vi "20110512 Plotter.vi"() -> ()   [LabVIEW 2009]
uses:
  <vilib>/Utility/miscctls.llb/LVPositionTypeDef.ctl
  <vilib>/Utility/tcp.llb/UDP Multicast Read-Only Open.vi
  shared programs/MySQL/Preset Query Enum.ctl
  <userlib>/_OpenG.lib/array/array.llb/Search 1D Array (String)__ogtk.vi
  <vilib>/Utility/miscctls.llb/LVRectTypeDef.ctl
panel:
  out "Mcast Data":string
  out "ScanStart ExptName":string
  out "TDMS file path":path
  out "Y Axis Default name":string
  in  "Tab Control 2":T1(tab)
  out "parameters to get":string[][](array[string])
  out "devices to get data from":string[](array[string])
  out "Axis Name List":string[](array[string])
  out "All Devices Core Info":string[][](array[string])
  out "Position 2":T2
  out "Position":T2
  out "UDP Mcast Error":errorcluster
  out "MY IP":string
  in  "Tab Control":enum32{"Main", "ShotData", "setup"}(tab)
  in  "Y Axis 2":u16(ring) items=["FakeCam1 shot #", "FakeCam1 exposure", "FakeCam1 gain", "Shot #"]
  in  "FilePath":bool
  out "xy graph":cluster{dbl[], dbl[]}[](graph)=[{[1.0, 2.0, 3.0, 4.0, 5.0, 6.0, 7.0, 8.0, 9.0, 10.0, 11.0, 12.0, 13.0, 14.0, 15.0, 16.0, 17.0, 18.0, 19.0, 20.0, 21.0, 22.0, 23.0, 24.0, 25.0, 26.0, 27.0, 28.0, 29.0, 30.0, 31.0, 32.0, 33.0, 34.0, 35.0, 36.0, 37.0, 38.0, 39.0, 40.0, 41.0, 42.0, 43.0, 44.0, 45.0, 46.0, 47.0, 48.0, 49.0, 50.0, 51.0, 52.0, 53.0, 54.0, 55.0, 56.0, 57.0, 58.0, 59.0, 60.0, 0.0, 0.0, 0.0], [0.1, 0.1, 0.1, 0.1, 0.1, 0.1, 0.1, 0.1, 0.1, 0.1, 0.1, 0.1, 0.1, 0.1, 0.1, 0.1, 0.1, 0.1, 0.1, 0.1, 0.15, 0.15, 0.15, 0.15, 0.15, 0.15, 0.15, 0.15, 0.15, 0.15, 0.15, 0.15, 0.15, 0.15, 0.15, 0.15, 0.15, 0.15, 0.15, 0.15, 0.2, 0.2, 0.2, 0.2, 0.2, 0.2, 0.2, 0.2, 0.2, 0.2, 0.2, 0.2, 0.2, 0.2, 0.2, 0.2, 0.2, 0.2, 0.2, 0.2, 0.0, 0.0, 0.0]}, {[1.0, 2.0, 3.0, 4.0, 5.0, 6.0, 7.0, 8.0, 9.0, 10.0, 11.0, 12.0, 13.0, 14.0, 15.0, 16.0, 17.0, 18.0, 19.0, 20.0, 21.0, 22.0, 23.0, 24.0, 25.0, 26.0, 27.0, 28.0, 29.0, 30.0, 31.0, 32.0, 33.0, 34.0, 35.0, 36.0, 37.0, 38.0, 39.0, 40.0, 41.0, 42.0, 43.0, 44.0, 45.0, 46.0, 47.0, 48.0, 49.0, 50.0, 51.0, 52.0, 53.0, 54.0, 55.0, 56.0, 57.0, 58.0, 59.0, 60.0, 0.0, 0.0, 0.0], [1.0, 2.0, 3.0, 4.0, 5.0, 6.0, 7.0, 8.0, 9.0, 10.0, 11.0, 12.0, 13.0, 14.0, 15.0, 16.0, 17.0, 18.0, 19.0, 20.0, 21.0, 22.0, 23.0, 24.0, 25.0, 26.0, 27.0, 28.0, 29.0, 30.0, 31.0, 32.0, 33.0, 34.0, 35.0, 36.0, 37.0, 38.0, 39.0, 40.0, 41.0, 42.0, 43.0, 44.0, 45.0, 46.0, 47.0, 48.0, 49.0, 50.0, 51.0, 52.0, 53.0, 54.0, 55.0, 56.0, 57.0, 58.0, 59.0, 60.0, 0.0, 0.0, 0.0]}]
  in  "Y Axis":u16(ring) items=["FakeCam1 shot #", "FakeCam1 exposure", "FakeCam1 gain"]
  in  "X Axis":u16(ring)=1 items=["FakeCam1 shot #", "FakeCam1 exposure", "FakeCam1 gain"]
  in  "OK Button":bool
  out "xy graph":cluster{dbl[], dbl[]}[](graph)=[{[5.5, 15.5, 25.5, 35.5, 45.5, 55.5, 0.0], [0.1, 0.1, 0.15, 0.15, 0.2, 0.2, 0.0]}, {[5.5, 5.5, nan, 15.5, 15.5, nan, 25.5, 25.5, nan, 35.5, 35.5, nan, 45.5, 45.5, nan, 55.5, 55.5, nan, 0.0, 0.0, nan], [0.1, 0.1, nan, 0.1, 0.1, nan, 0.15, 0.15, nan, 0.15, 0.15, nan, 0.2, 0.2, nan, 0.2, 0.2, nan, 0.0, 0.0, nan]}, {[5.5, 15.5, 25.5, 35.5, 45.5, 55.5, 0.0], [5.5, 15.5, 25.5, 35.5, 45.5, 55.5, 0.0]}, {[5.5, 5.5, nan, 15.5, 15.5, nan, 25.5, 25.5, nan, 35.5, 35.5, nan, 45.5, 45.5, nan, 55.5, 55.5, nan, 0.0, 0.0, nan], [3.0, 8.0, nan, 13.0, 18.0, nan, 23.0, 28.0, nan, 33.0, 38.0, nan, 43.0, 48.0, nan, 53.0, 58.0, nan, 0.0, 0.0, nan]}]
  in  "Fixed Interval":bool
  in  "Interval":dbl format="%.3p"
  in  "Auto Interval":bool
  in  "Error Bar Type":T3(ring)
  in  "Experiment":u16(ring) items=["10TW colliding pulse", "FakeCam1only", "TREX high power", "TREX low power"]
  out "Current State":string
  out "Mcast Path Data":string
  in  "replot":bool
  in  "file path":path
  out "Path used":path
  out "device data Spreadsheet format":string[][](array[string])
  in  "Left":i16=25
  in  "Top":i16=75
  out "x axis name":string
  # "C:\\Documents and Settings\\loasis\\My Documents\\test to delete\\scans\\Scan008\\Scan008.tdms"
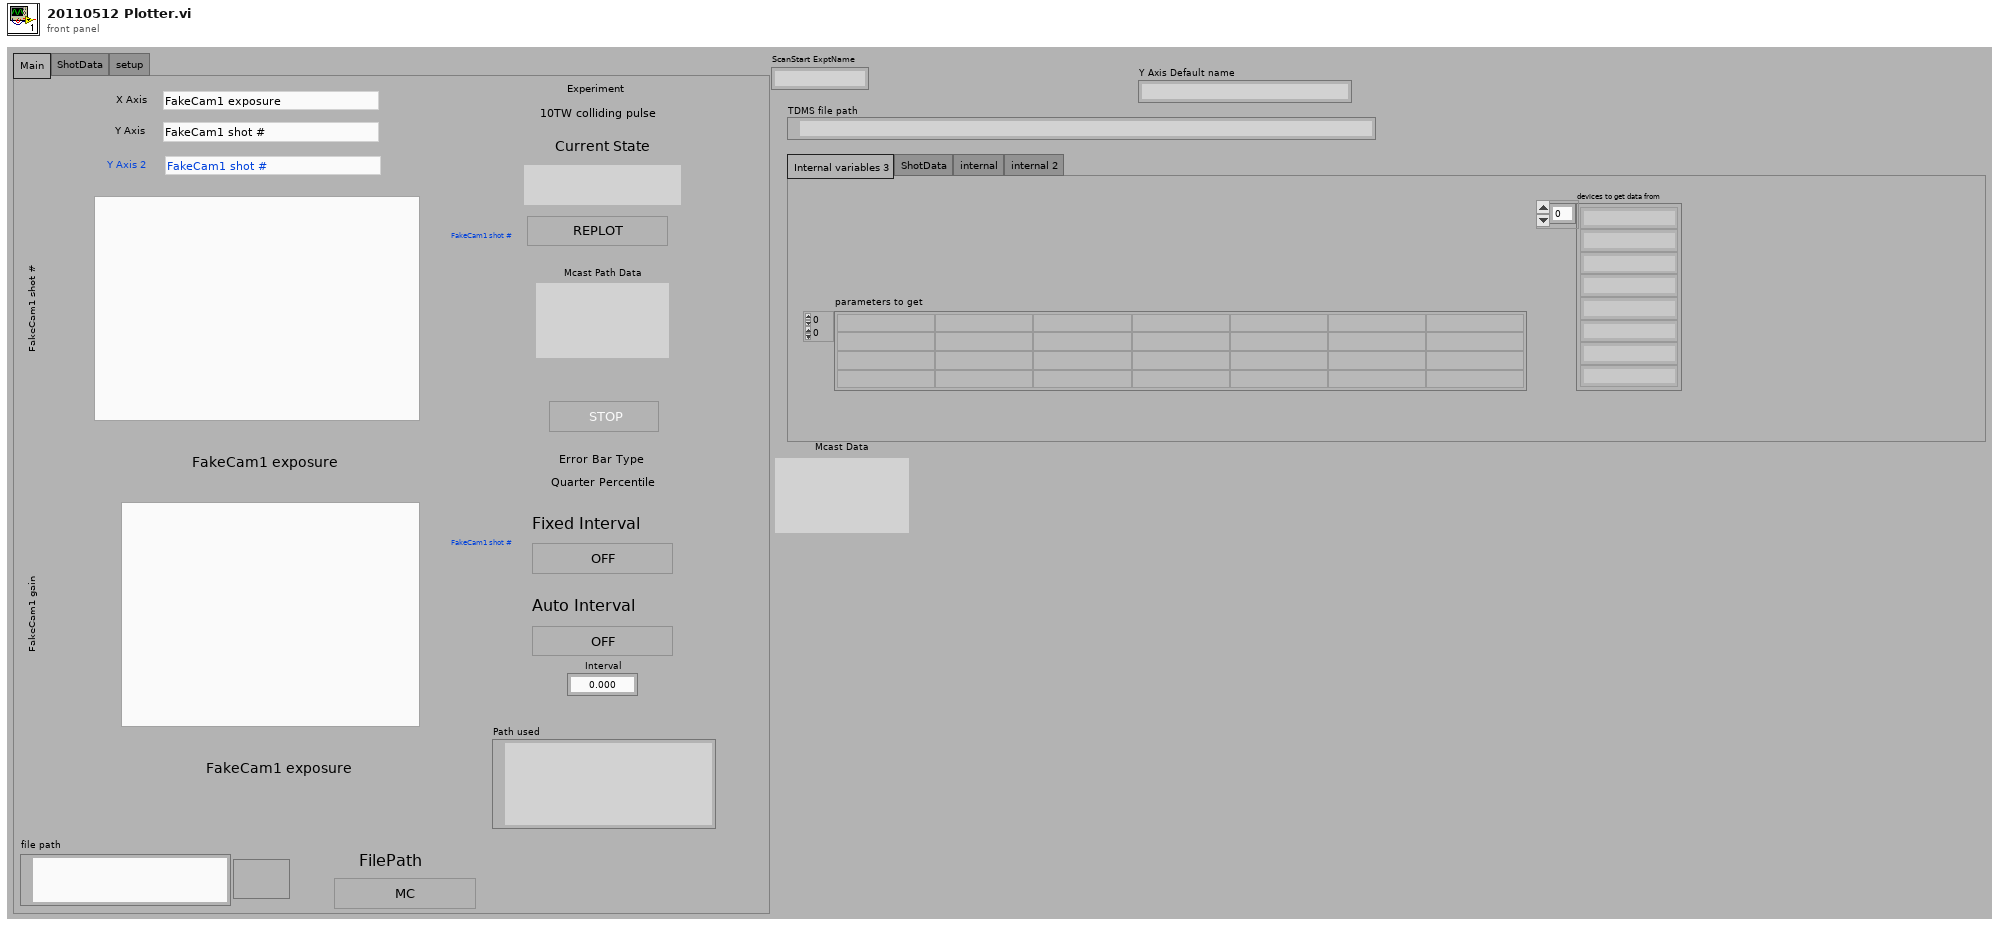
[diagram p1: front panel]
types:
  T1 = enum32{"Internal variables 3", "ShotData", "internal", "internal 2"}
  T2 = typedef "LVPositionTypeDef.ctl" = cluster{"Left":i32, "Top":i32}
  T3 = enum16{"Quarter Percentile", "Standard Deviation"}
  T4 = enum32{"invalid app kind", "Development System", "Run Time System", "Student Edition", "Embedded LabVIEW", "Evaluation", "Custom"}
  T5 = enum32{"Invalid", "Standard", "Closed", "Hidden", "Minimized", "Maximized"}
  T6 = typedef "Preset Query Enum.ctl" = enum16{"Get Locations", "Get classes", "Get expt variables to set at scanstart for particular device", "Get expt devices and variables with start values", "Get expt devices and variables (with data to get)", "Get expt devices with data to get", "Get Expt devices", "Get all devices basic properties", "Get Expt names", "Get MultiCast IP of experiment", "Get MC Ports", "Get device network comm port", "Get basic device properties", "Get all setable variables of a device", "Get all variables of a devicetype", "Get all variables of a device", "Get all devices"}
  T7 = typedef "LVRectTypeDef.ctl" = cluster{"Left":i16, "Top":i16, "Right":i16, "Bottom":i16}
  T8 = enum16{"open", "open or create", "create or replace", "create", "open (read-only)"}
  T9 = cluster{"Ring Refnum x":refnum<vi>, "Ring Refnum y":refnum<vi>, "Ring Refnum y 2":refnum<vi>, "XY Graph Refnum":refnum<vi>}
  T10 = cluster{"Core":cluster{"Current VI Reference":refnum<vi>, "Close Panel on Exit?":bool}, "Variable selector":u16, "variable parameters":string[], "list of variables":string[], "UDP Command to send":string, "Device List":string[], "Config path":path, "Devices Selector":u16, "Device Config file array":string[][], "All Devices Core Info":string[][], "Location Filter":u16, "Filtered Device List":string[], "Class Filter":u16, "Command to Send":string, "Devices Path":path, "UDP ID":refnum<k16>, "parameter vals scanned":dbl[], "List Commands Not Executed":string[], "Expected slow response":string, "MCast Address":string, "MCast Local Port":u16, "MCast Remote Port":u16, "UDP timeout ms":i32, "Scan Number":i32, "Shot Number":i32, "Scan Data Titles":string[], "Scan Data Array":dbl[], "Expt Config Files":string[], "Experiment name":string, "UDP fast port":u16, "name":string, "ScanData to receive":string[][], "UDP Listen Ports":u16[], "Device Names for scan data":string[], "ShotData":string[], "Scans Path":path, "Device xxx Path":path, "numeric?":bool, "Last Slow response":string, "Mcast command":string, "Device Status Array":bool[], "expt config file array":string[][], "Shot Data plotter":string[][], "Data titles from config array":string[], "TDMS file path":path}
  T11 = typedef "LVPointTypeDef.ctl" = cluster{"Horizontal":i16, "Vertical":i16}
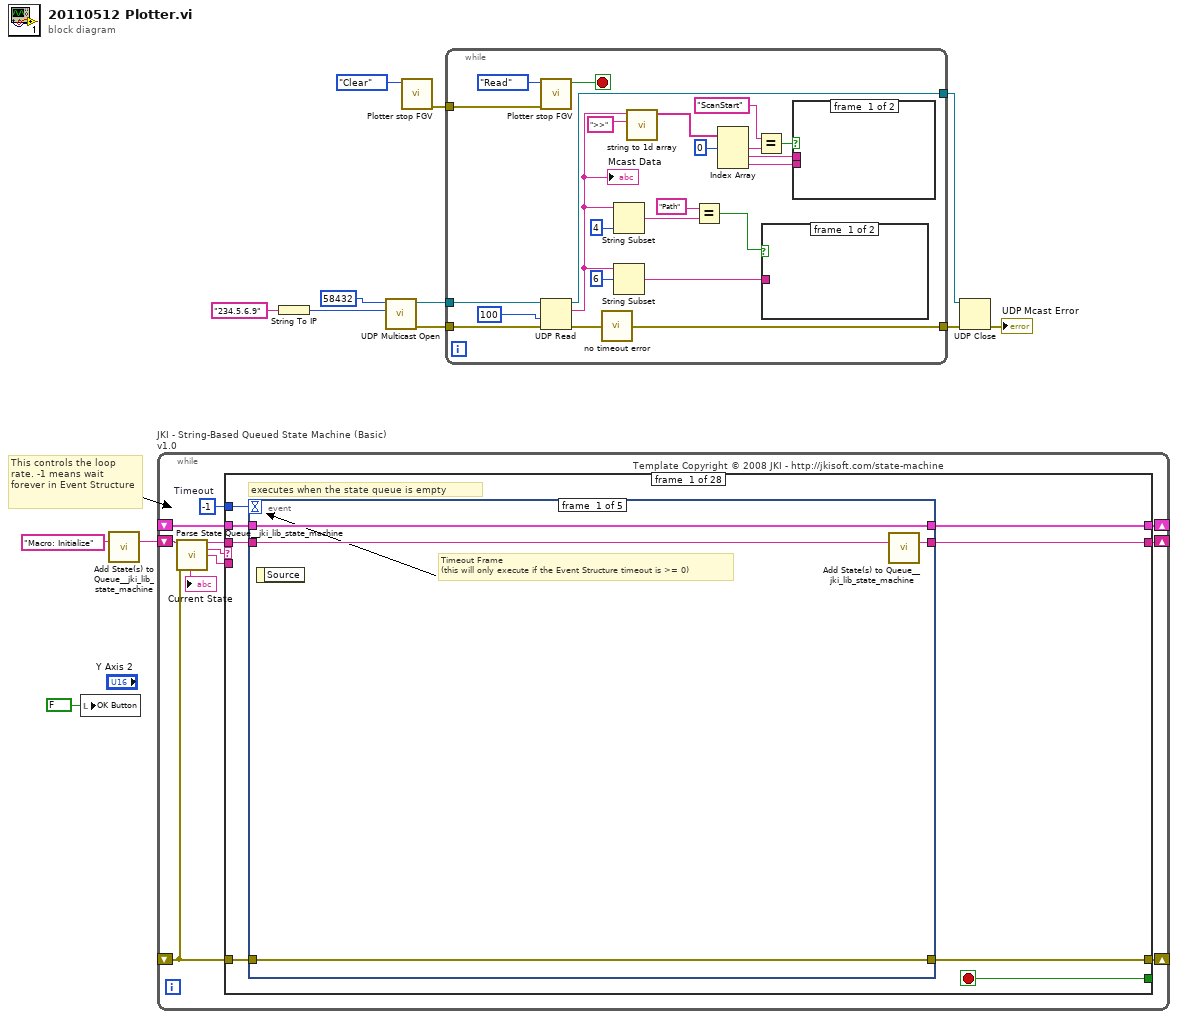
[diagram p0: block diagram]
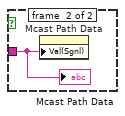
[diagram p2: hidden frame]
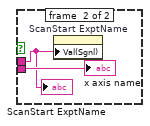
[diagram p3: hidden frame]
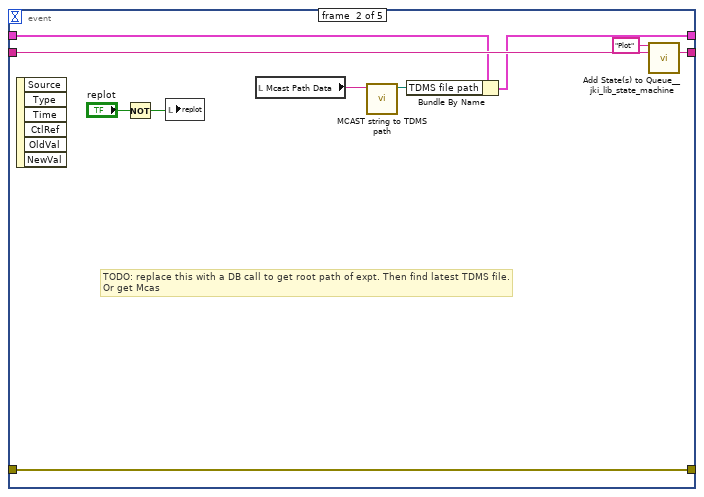
[diagram p4: hidden frame]
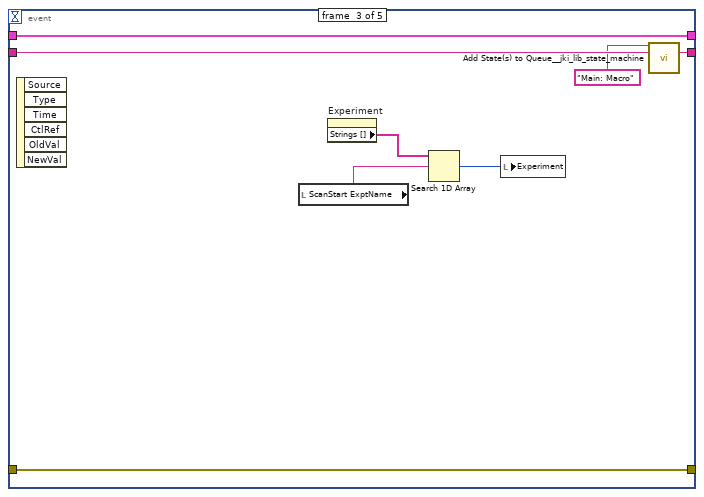
[diagram p5: hidden frame]
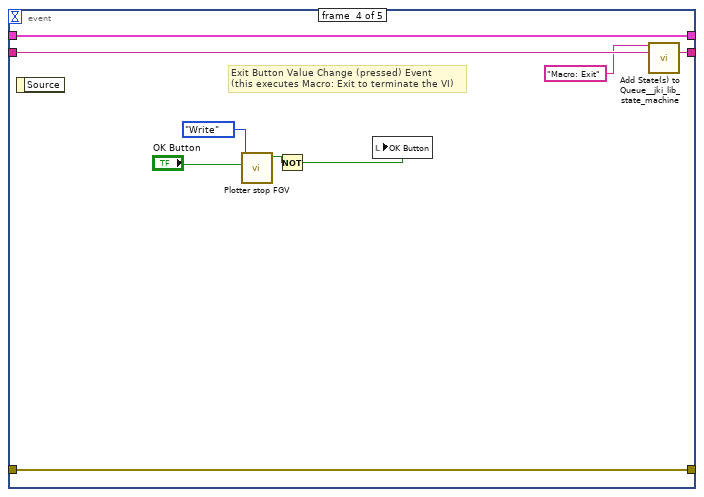
[diagram p6: hidden frame]
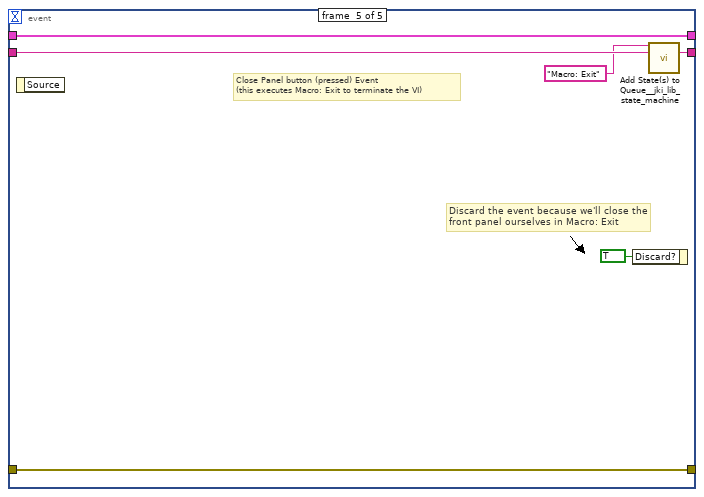
[diagram p7: hidden frame]
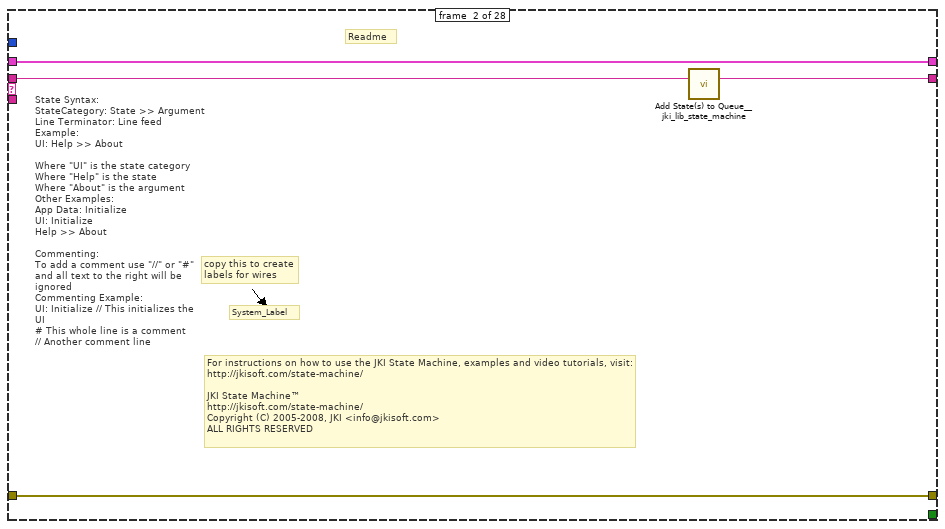
[diagram p8: hidden frame]
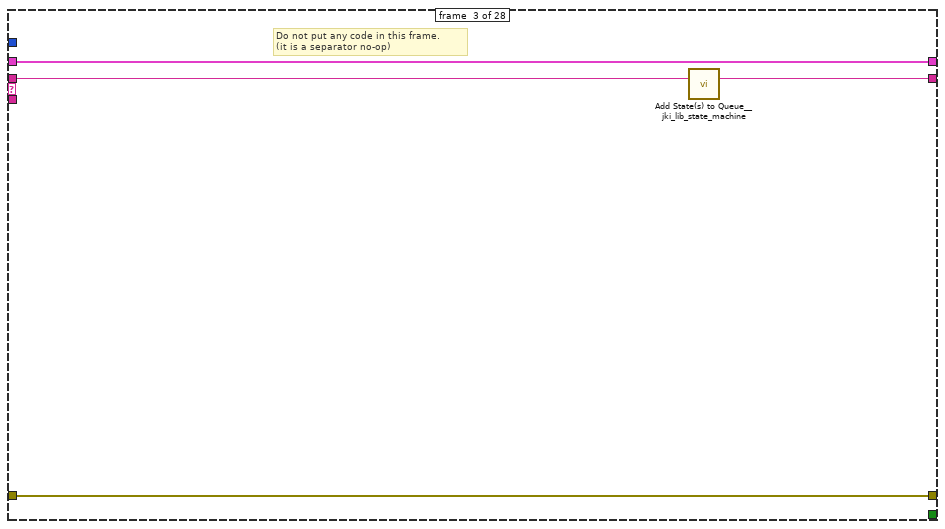
[diagram p9: hidden frame]
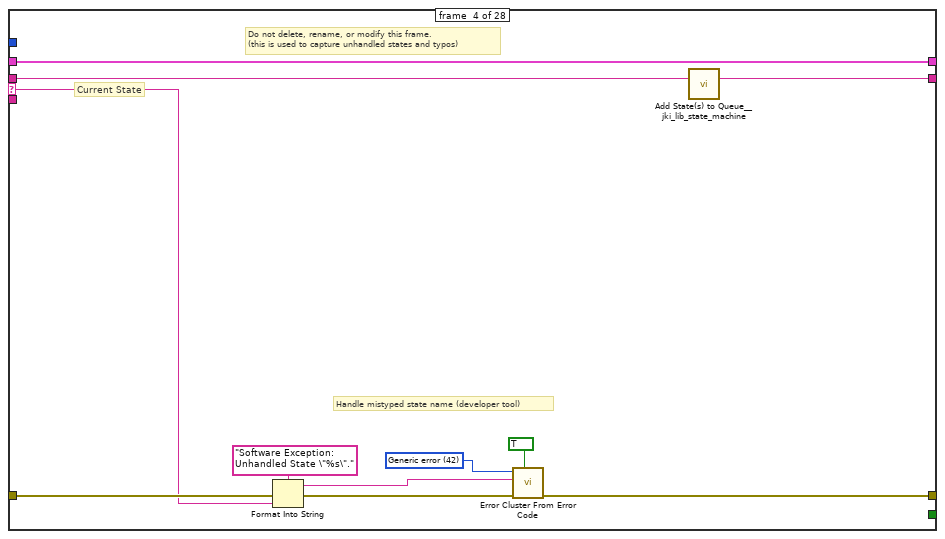
[diagram p10: hidden frame]
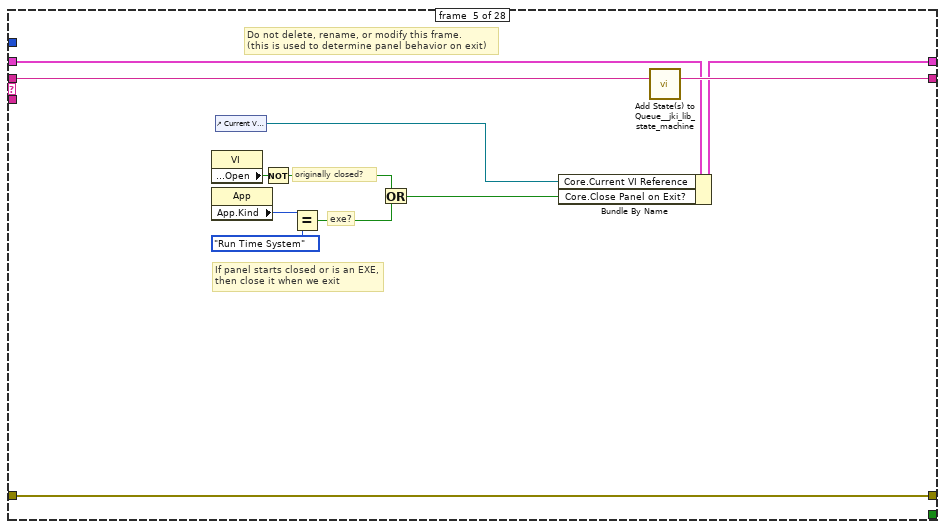
[diagram p11: hidden frame]
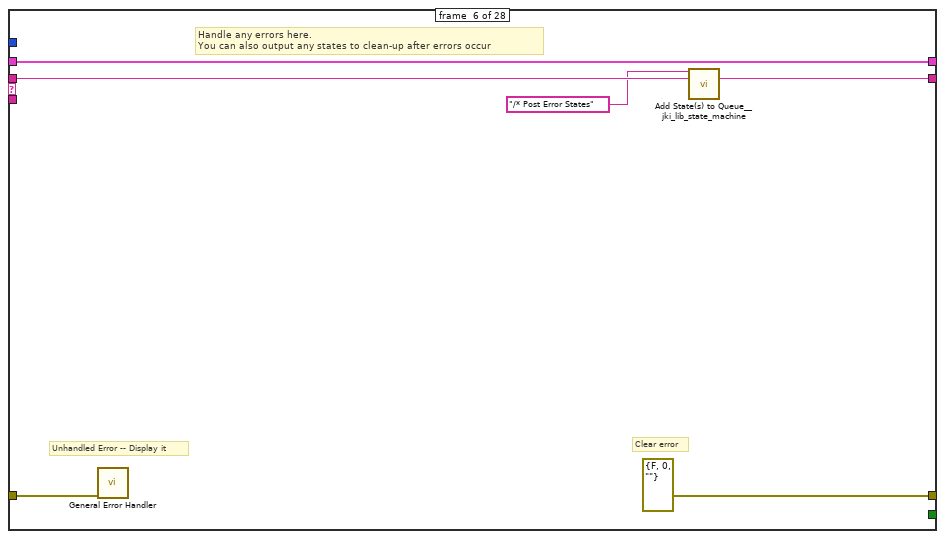
[diagram p12: hidden frame]
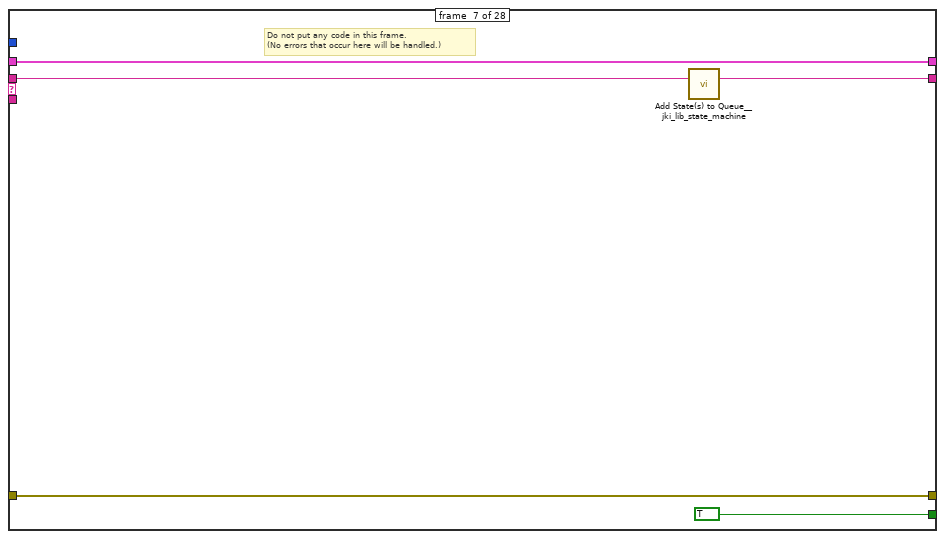
[diagram p13: hidden frame]
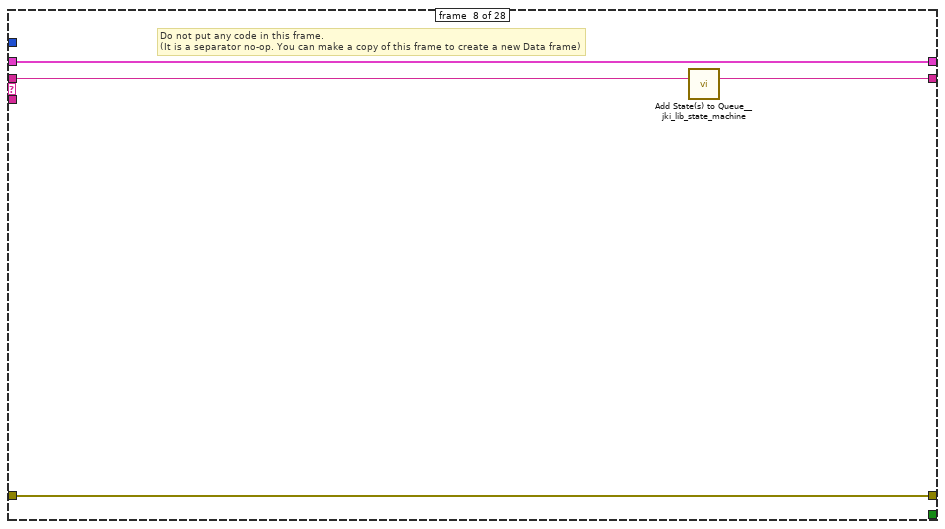
[diagram p14: hidden frame]
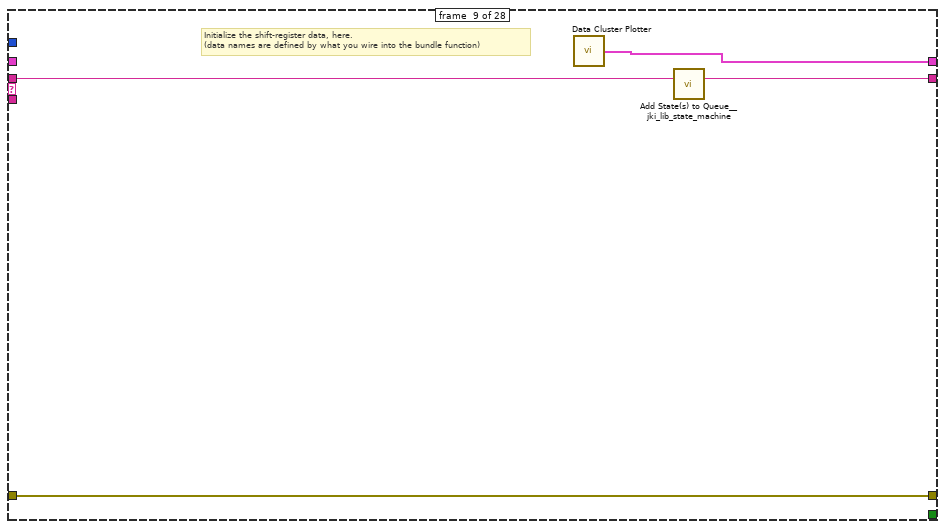
[diagram p15: hidden frame]
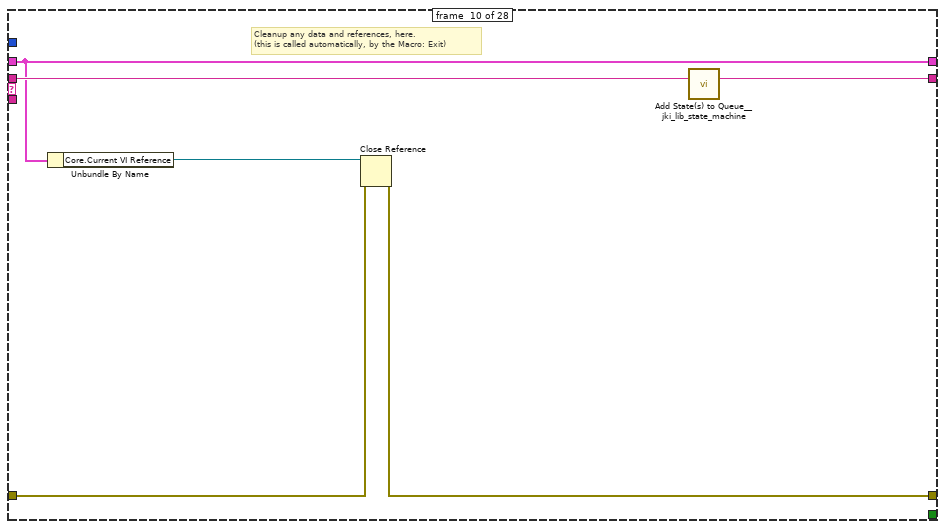
[diagram p16: hidden frame]
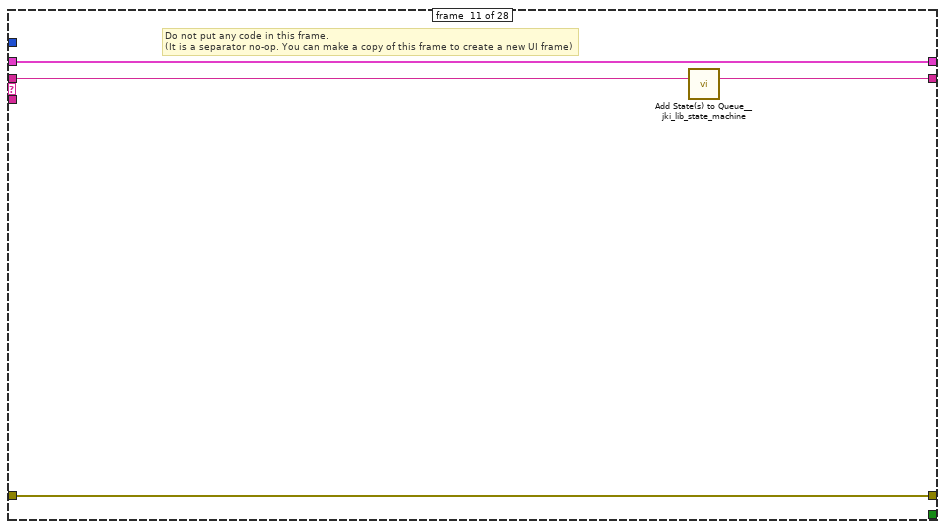
[diagram p17: hidden frame]
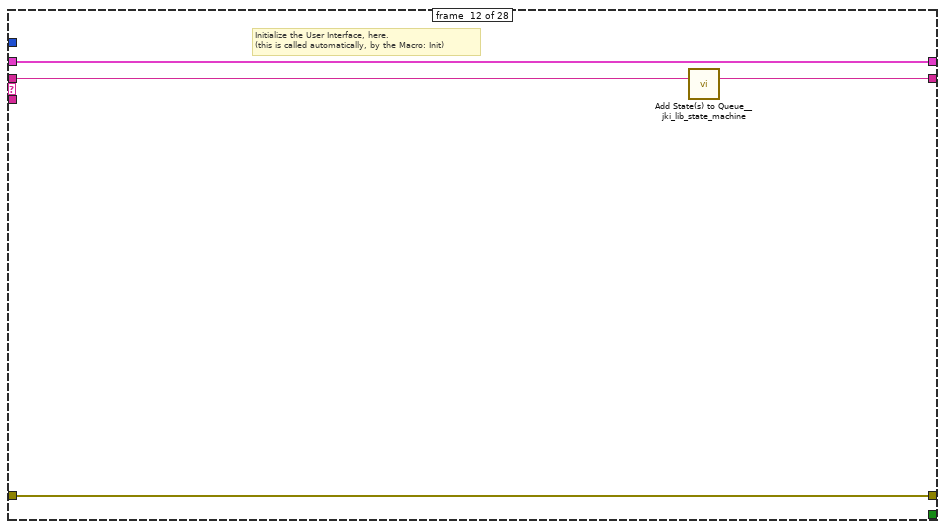
[diagram p18: hidden frame]
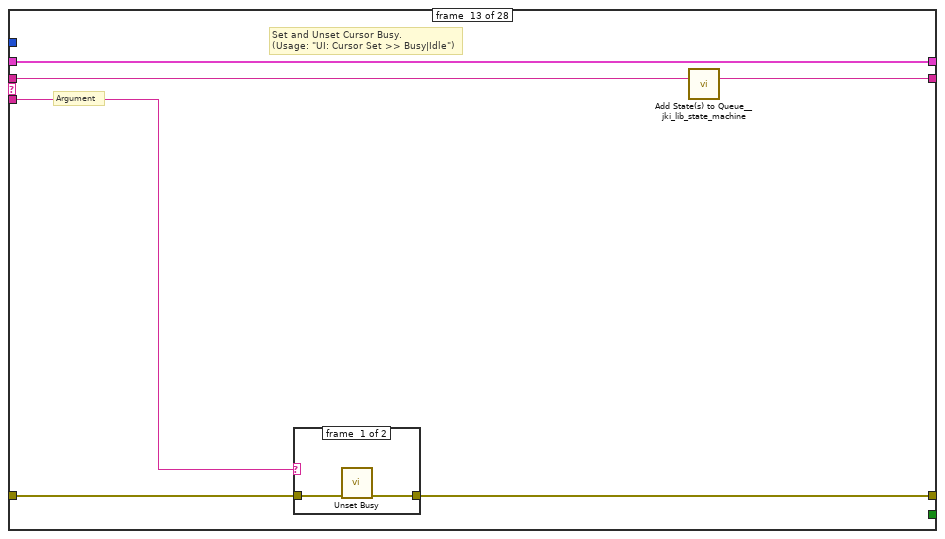
[diagram p19: hidden frame]
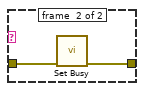
[diagram p20: hidden frame]
diagram:
  # "This controls the loop rate. -1 means wait forever in Event Structure"
  n1 = local write "OK Button"(FALSE ("OK Button")) -> ()
  n2 = call <vilib>:"Add State(s) to Queue__jki_lib_state_machine.vi"("State(s) in (\"\")"="Macro: Initialize") -> ("States Out"=w13:string)  [unwired: 14 in]
  n3 = while "JKI - String-Based Queued State Machine (Basic) v1.0" {
    shift-right: [w17] -> _
    shift-left: _ -> [w16]
    shift-right: [w20] -> _
    shift-left: _ -> [w14]
    shift-right: [w19] -> _
    shift-left: w13 -> [w21]
    stop <- w18 stop-if-true
    w15 = -1  # Timeout
    # "Template Copyright © 2008 JKI - http://jkisoft.com/state-machine"
    n4 = call <vilib>:"Parse State Queue__jki_lib_state_machine.vi"("State Queue"=w21, "Error In (no error)"=w14) -> ("Remaining States"=w23:string, "Current State"=w24:string, "Arguments"=w22:string)  [unwired: 11 in]
    "Current State" <- w24
    n5 = case shown="\"\", \"Idle\"" w24 {
      selector: w24 -> [_ _ _ w77 _ _ _ _ _ _ _ _ _ _ _ _ _ _ _ _ _ _ _ _ _ _ _ _]
      tunnel: w23 -> [w31 w72 w76 w81 w99 w105 w110 w114 w118 w124 w128 w132 w138 w149 w175 w180 w190 w194 w200 w209 w217 w233 w244 w266 w297 w304 w308 w362]
      tunnel: w22 -> [_ _ _ _ _ _ _ _ _ _ _ _ w133 w143 _ _ _ _ _ _ _ _ _ _ _ _ _ _]
      tunnel: w16 -> [w29 w69 w73 w79 w90 w102 w108 w111 _ w119 w125 w130 w136 w145 w172 w176 w188 w191 w197 w206 w215 w231 w235 w255 w294 w300 w305 w359]
      tunnel: [w28 w70 w74 w83 w96 errorcluster {"status"=FALSE, "code"=0, "source"=""} ("error out") w107 w112 w116 w120 w126 w129 w134 w146 w173 w178 w181 w192 w198 w201 w212 w220 w242 w264 w295 w302 w306 w360] -> w20
      tunnel: w14 -> [w27 w70 w74 w82 w96 w101 w107 w112 w116 w121 w126 w129 w135 w147 w173 w178 w181 w192 w198 w202 w212 w221 w242 w264 w295 w302 w306 w360]
      tunnel: [w30 w71 w75 w80 w98 w104 w109 w113 w117 w123 w127 w131 w137 w148 w174 w179 w189 w193 w199 w208 w216 w232 w243 w265 w296 w303 w307 w361] -> w19
      tunnel: [_ _ _ _ _ _ TRUE _ _ _ _ _ _ _ _ _ _ _ _ _ _ _ _ _ _ _ _ _] -> w18
      tunnel: [w26 w69 w73 w79 w97 w102 w108 w111 w115 w119 w125 w130 w136 w145 w172 w176 w188 w191 w197 w205 w214 w230 w234 w255 w294 w301 w305 w359] -> w17
      tunnel: w15 -> [w25 _ _ _ _ _ _ _ _ _ _ _ _ _ _ _ _ _ _ _ _ _ _ _ _ _ _ _]
      frame #0 {
        # "executes when the state queue is empty"
        n6 = event shown="[2] \"ScanStart ExptName\": Value Change" {
          selector: _ -> [_ _ _ _ _]
          dyn-events: _ -> [_ _ _ _ _]
          timeout: w25 -> [_ _ _ _ _]
          tunnel: w31 -> [w35 w45 w53 w62 w68]
          tunnel: [w34 w44 w52 w61 w67] -> w30
          tunnel: w29 -> [w32 w41 w49 w59 w65]
          tunnel: [w33 w43 w51 w60 w66] -> w28
          tunnel: w27 -> [w33 w43 w51 w60 w66]
          tunnel: [w32 w40 w49 w59 w65] -> w26
          event #0 {
            # "Timeout Frame\n(this will only execute if the Event Structure timeout is >= 0)"
            n7 = event-data() -> ()  [unwired: 1 in, 1 out]
            n8 = call <vilib>:"Add State(s) to Queue__jki_lib_state_machine.vi"("State(s) in (\"\")"=w35) -> ("States Out"=w34:string)  [unwired: 14 in]
          }
          event #1 {
            # "TODO: replace this with a DB call to get root path of expt. Then find latest TDMS file.\nOr get Mcas"
            n9 = event-data() -> ()  [unwired: 1 in, 6 out]
            n10 = Not(x="replot") -> (.not. x?=w38:bool)
            n11 = local write "replot"(w38) -> ()
            n12 = local read "Mcast Path Data"() -> (w37:string)
            n13 = call "MCAST string to TDMS path.vi"("MCAST path"=w37) -> ("TDMS path"=w36:path)  [unwired: 10 in]
            n14 = Bundle By Name(cluster=w41, "TDMS file path"=w36) -> (w40:T10)
            n15 = call <vilib>:"Add State(s) to Queue__jki_lib_state_machine.vi"("State(s) in Front (\"\")"="Plot" ("State(s) in Front (\"\")"), "State(s) in (\"\")"=w45) -> ("States Out"=w44:string)  [unwired: 13 in]
          }
          event #2 {
            n16 = event-data() -> ()  [unwired: 1 in, 6 out]
            n17 = local read "ScanStart ExptName"() -> (w47:string)
            n18 = property on="Experiment" class="Ring (strict)"() -> ("Strings []"=w48:string[])  [unwired: 2 in, 2 out]
            n19 = Search 1D Array(1D array=w48, element=w47) -> (index of element=w46:i32)  [unwired: 1 in]
            n20 = local write "Experiment"(w46) -> ()
            n21 = call <vilib>:"Add State(s) to Queue__jki_lib_state_machine.vi"("State(s) in Front (\"\")"="Main: Macro", "State(s) in (\"\")"=w53) -> ("States Out"=w52:string)  [unwired: 13 in]
          }
          event #3 {
            # "Exit Button Value Change (pressed) Event\n(this executes Macro: Exit to terminate the VI)"
            n22 = event-data() -> ()  [unwired: 1 in, 1 out]
            n23 = call "Plotter stop FGV.vi"("Stop in"="OK Button", "Function"=enum16{"Read", "Write", "Clear"}."Write") -> ("Stop out"=w56:bool)  [unwired: 8 in, 1 out]
            n24 = Not(x=w56) -> (.not. x?=w55:bool)
            n25 = local write "OK Button"(w55) -> ()
            n26 = call <vilib>:"Add State(s) to Queue__jki_lib_state_machine.vi"("State(s) in Front (\"\")"="Macro: Exit", "State(s) in (\"\")"=w62) -> ("States Out"=w61:string)  [unwired: 13 in]
          }
          event #4 {
            # "Discard the event because we'll close the front panel ourselves in Macro: Exit"
            # "Close Panel button (pressed) Event\n(this executes Macro: Exit to terminate the VI)"
            n27 = event-data() -> ()  [unwired: 1 in, 1 out]
            n28 = event-data("Discard?"=TRUE) -> ()  [unwired: 1 in, 1 out]
            n29 = call <vilib>:"Add State(s) to Queue__jki_lib_state_machine.vi"("State(s) in Front (\"\")"="Macro: Exit", "State(s) in (\"\")"=w68) -> ("States Out"=w67:string)  [unwired: 13 in]
          }
        }
      }
      frame #1 {
        # "For instructions on how to use the JKI State Machine, examples and video tutorials, visit:\nhttp://jkisoft.com/state-machine/\n\nJKI State Machine™\nhttp://jkisoft.com/state-machine/\nCopyright (C) 2005-2008, JKI <info@jkisoft.com>\nALL RIGHTS RESERVED"
        # "copy this to create labels for wires"
        # "System_Label"
        # "State Syntax:\nStateCategory: State >> Argument\nLine Terminator: Line feed\nExample:\nUI: Help >> About\n\nWhere \"UI\" is the state category\nWhere \"Help\" is the state\nWhere \"About\" is the argument\nOther Examples:\nApp Data: Initialize\nUI: Initialize\nHelp >> About\n\nCommenting:\nTo add a comment use \"//\" or \"#\" and all text to the right will be ignored\nCommenting Example:\nUI: Initialize // This initializes the UI\n# This whole line is a comment\n// Another comment line"
        # "Readme"
        n30 = call <vilib>:"Add State(s) to Queue__jki_lib_state_machine.vi"("State(s) in (\"\")"=w72) -> ("States Out"=w71:string)  [unwired: 14 in]
      }
      frame #2 {
        # "Do not put any code in this frame.\n(it is a separator no-op)"
        n31 = call <vilib>:"Add State(s) to Queue__jki_lib_state_machine.vi"("State(s) in (\"\")"=w76) -> ("States Out"=w75:string)  [unwired: 14 in]
      }
      frame #3 {
        w86 = 42 items=["No error", "Argument error", "Memory is full", "Out of zone", "End of file", "File already open", "Generic file I/O error", "File not found", "File permission error", "Disk is full", "Duplicate path", "Too many files open", "System feature not enabled", "Resource file not found", "Cannot add resource", "Resource not found", "Image not found", "Image memory error", "Pen does not exist", "Config type invalid", "Config token not found", "Config parse error", "Config memory error", "Bad external code format", "Bad external code offset", "External code not present", "Null window", "Destroy window error", "Null menu", "Print aborted", "Bad print record", "Print driver error", "Windows error during printing", "Memory error during printing", "Print dialog error", "Generic print error", "Invalid device refnum", "Device not found", "Device parameter error", "Device unit error", "Cannot open device", "Device call aborted", "Generic error", "Cancelled by user", "Object ID too low", "Object ID too high", "Object not in heap", "Unknown heap", "Unknown object (invalid DefProc)", "Unknown object (DefProc not in table)", "Message out of range", "Invalid (null) method", "Unknown message", "Manager call not supported", "Bad address", "Network operation in progress", "Network operation timed out", "Connection is busy", "Network attribute not supported", "Network error", "Address in use", "System out of memory", "Connection aborted", "Connection refused", "Not connected", "Already connected", "Connection closed", "Initialization error (interapplication manager)", "Bad occurrence", "Wait on unbound occurrence handler", "Occurrence queue overflow", "Datalog type conflict", "Unused", "Unrecognized type (interapplication manager)", "Memory corrupt", "Failed to make temporary DLL", "Old CIN version", "Drag socket not found", "Failed to load drop-object", "Failed to register OLE object", "Failed to release OLE object", "Format specifier type mismatch", "Unknown format specifier", "Too few format specifiers", "Too many format specifiers", "Scan failed", "Newer CIN version", "Error converting to variant", "Runtime menu error", "Password tampered", "Variant attribute not found", "Incompatible variant data type", "Event data is not available", "Event Store is not present", "Occurrence is not found", "Event Queue is not created", "Event info is not available", "Refnum passed is NULL", "Error retrieving Class GUID", "Error retrieving CoClass GUID", "Error retrieving TypeLib GUID.", "Bad built application magic bytes.", "Specific driver is different from the specific driver associated with the Logical Name.", "There is no session opened to the class driver.", "Max Error", "MAX - Error with config objects", "MAX - Error loading configuration", "MAX - Group not supported"]
        # "Current State"
        # "Do not delete, rename, or modify this frame.\n(this is used to capture unhandled states and typos)"
        # "Handle mistyped state name (developer tool)"
        n32 = Format Into String(format string="Software Exception: Unhandled State \"%s\"." ("message"), error in=w82, w77) -> (resulting string=w85:string, error out=w84:errorcluster)  [unwired: 1 in]
        n33 = call <vilib>:"Error Cluster From Error Code.vi"("show call chain? (False)"=TRUE, "error in (no error)"=w84, "error message (\"\")"=w85, "error code (0)"=w86) -> ("error out"=w83:errorcluster)  [unwired: 5 in]
        n34 = call <vilib>:"Add State(s) to Queue__jki_lib_state_machine.vi"("State(s) in (\"\")"=w81) -> ("States Out"=w80:string)  [unwired: 14 in]
      }
      frame #4 {
        # "Do not delete, rename, or modify this frame.\n(this is used to determine panel behavior on exit)"
        # "originally closed?"
        # "exe?"
        # "If panel starts closed or is an EXE, then close it when we exit"
        n35 = property class="VI"() -> ("Front Panel.Open"=w95:bool)  [unwired: 2 in, 2 out]
        n36 = property class="App"() -> ("App.Kind"=w94:T4)  [unwired: 2 in, 2 out]
        n37 = control-ref of="Current VI Reference"() -> (w88:refnum<vi>)
        n38 = Not(x=w95) -> (.not. x?=w92:bool)
        n39 = Equal?(x=w94, y=T4."Run Time System" ("Application:Kind")) -> (x = y?=w91:bool)
        n40 = Or(x=w92, y=w91) -> (x .or. y?=w89:bool)
        n41 = Bundle By Name(cluster=w90, "Core.Current VI Reference"=w88, "Core.Close Panel on Exit?"=w89) -> (w97:T10)
        n42 = call <vilib>:"Add State(s) to Queue__jki_lib_state_machine.vi"("State(s) in (\"\")"=w99) -> ("States Out"=w98:string)  [unwired: 14 in]
      }
      frame #5 {
        # "Unhandled Error -- Display it"
        # "Handle any errors here.\nYou can also output any states to clean-up after errors occur"
        # "Clear error"
        n43 = call <vilib>:"General Error Handler.vi"("error in (no error)"=w101) -> ()  [unwired: 10 in, 5 out]
        n44 = call <vilib>:"Add State(s) to Queue__jki_lib_state_machine.vi"("State(s) in Front (\"\")"="/* Post Error States", "State(s) in (\"\")"=w105) -> ("States Out"=w104:string)  [unwired: 13 in]
      }
      frame #6 {
        # "Do not put any code in this frame.\n(No errors that occur here will be handled.)"
        n45 = call <vilib>:"Add State(s) to Queue__jki_lib_state_machine.vi"("State(s) in (\"\")"=w110) -> ("States Out"=w109:string)  [unwired: 14 in]
      }
      frame #7 {
        # "Do not put any code in this frame.\n(It is a separator no-op. You can make a copy of this frame to create a new Data frame)"
        n46 = call <vilib>:"Add State(s) to Queue__jki_lib_state_machine.vi"("State(s) in (\"\")"=w114) -> ("States Out"=w113:string)  [unwired: 14 in]
      }
      frame #8 {
        # "Initialize the shift-register data, here.\n(data names are defined by what you wire into the bundle function)"
        n47 = call "Data Cluster Plotter.vi"() -> ("output cluster"=w115:T10)
        n48 = call <vilib>:"Add State(s) to Queue__jki_lib_state_machine.vi"("State(s) in (\"\")"=w118) -> ("States Out"=w117:string)  [unwired: 14 in]
      }
      frame #9 {
        # "Cleanup any data and references, here.\n(this is called automatically, by the Macro: Exit)"
        n49 = Unbundle By Name(w119) -> ("Core.Current VI Reference"=w122:refnum<vi>)
        n50 = Close Reference(reference=w122, error in (no error)=w121) -> (error out=w120:errorcluster)
        n51 = call <vilib>:"Add State(s) to Queue__jki_lib_state_machine.vi"("State(s) in (\"\")"=w124) -> ("States Out"=w123:string)  [unwired: 14 in]
      }
      frame #10 {
        # "Do not put any code in this frame.\n(It is a separator no-op. You can make a copy of this frame to create a new UI frame)"
        n52 = call <vilib>:"Add State(s) to Queue__jki_lib_state_machine.vi"("State(s) in (\"\")"=w128) -> ("States Out"=w127:string)  [unwired: 14 in]
      }
      frame #11 {
        # "Initialize the User Interface, here.\n(this is called automatically, by the Macro: Init)"
        n53 = call <vilib>:"Add State(s) to Queue__jki_lib_state_machine.vi"("State(s) in (\"\")"=w132) -> ("States Out"=w131:string)  [unwired: 14 in]
      }
      frame #12 {
        # "Argument"
        # "Set and Unset Cursor Busy.\n(Usage: \"UI: Cursor Set >> Busy|Idle\")"
        n54 = case shown="\"Idle\", Default" w133 {
          tunnel: w135 -> [w140 w142]
          tunnel: [w139 w141] -> w134
          frame #0 {
            n55 = call <vilib>:"Unset Busy.vi"("error in (no error)"=w140) -> ("error out"=w139:errorcluster)  [unwired: 10 in]
          }
          frame #1 {
            n56 = call <vilib>:"Set Busy.vi"("error in (no error)"=w142) -> ("error out"=w141:errorcluster)  [unwired: 9 in, 1 out]
          }
        }
        n57 = call <vilib>:"Add State(s) to Queue__jki_lib_state_machine.vi"("State(s) in (\"\")"=w138) -> ("States Out"=w137:string)  [unwired: 14 in]
      }
      frame #13 {
        # "Argument"
        # "Set Front Panel Open or Closed\n(Usage: \"UI: Front Panel State >> Open|Close\")"
        n58 = Unbundle By Name(w145) -> ("Core.Current VI Reference"=w144:refnum<vi>)
        n59 = case shown="\"Open\", Default" w143 {
          tunnel: w147 -> [w153 w166]
          tunnel: [w155 w167] -> w146
          tunnel: w144 -> [w154 w164]
          frame #0 {
            n60 = property class="VI"(reference=w154, error in=w153) -> (reference out=w151:refnum<vi>, error out=w152:errorcluster, "Front Panel.Open"=w150:bool)
            n61 = case shown="True" w150 {
              tunnel: [w158 w161] -> w155
              tunnel: w152 -> [w157 w161]
              tunnel: w151 -> [w156 _]
              frame #0 {
                n62 = invoke class="VI" method="FP.Open"(reference=w156, error in=w157, "Activate"=TRUE, "State"=T5."Standard") -> (error out=w158:errorcluster)  [unwired: 1 in, 4 out]
              }
              frame #1 {
              }
            }
          }
          frame #1 {
            n63 = property class="VI"(reference=w164, error in=w166) -> (reference out=w163:refnum<vi>, error out=w165:errorcluster, "Front Panel.Open"=w162:bool)
            n64 = case shown="True" w162 {
              tunnel: [w168 w171] -> w167
              tunnel: w165 -> [w168 w170]
              tunnel: w163 -> [_ w169]
              frame #0 {
              }
              frame #1 {
                n65 = invoke class="VI" method="FP.Close"(reference=w169, error in=w170) -> (error out=w171:errorcluster)  [unwired: 1 in, 2 out]
              }
            }
          }
        }
        n66 = call <vilib>:"Add State(s) to Queue__jki_lib_state_machine.vi"("State(s) in (\"\")"=w149) -> ("States Out"=w148:string)  [unwired: 14 in]
      }
      frame #14 {
        # "Do not put any code in this frame.\n(It is a separator no-op. You can make a copy of this frame to create a new Macro frame)"
        n67 = call <vilib>:"Add State(s) to Queue__jki_lib_state_machine.vi"("State(s) in (\"\")"=w175) -> ("States Out"=w174:string)  [unwired: 14 in]
      }
      frame #15 {
        w177 = "Data: Initialize\nInitialize Core Data\nUI: Initialize\nUI: Front Panel State >> Open\nMain: Macro"  # Data: Initialize Initialize Core Data UI: Initialize UI: Front Panel State >> Open Main: Macro
        # "Initialization Macro\n(This is called once, when the VI starts)"
        n68 = call <vilib>:"Add State(s) to Queue__jki_lib_state_machine.vi"("State(s) in Front (\"\")"=w177, "State(s) in (\"\")"=w180) -> ("States Out"=w179:string)  [unwired: 13 in]
      }
      frame #16 {
        # "Exit Macro\n(This is called once, when the VI exits)"
        n69 = Unbundle By Name(w188) -> ("Core.Close Panel on Exit?"=w187:bool)
        n70 = Select(t="UI: Front Panel State >> Close", s=w187, f="") -> (s? t:f=w184:string)
        n71 = call <vilib>:"Add State(s) to Queue__jki_lib_state_machine.vi"("State(s) in (\"\")"=w184, "State(s) at Back (\"\")"="Data: Cleanup\nExit") -> ("States Out"=w182:string)  [unwired: 13 in]
        n72 = call <vilib>:"Add State(s) to Queue__jki_lib_state_machine.vi"("State(s) in Front (\"\")"=w182, "State(s) in (\"\")"=w190) -> ("States Out"=w189:string)  [unwired: 13 in]
      }
      frame #17 {
        # "Template Separator\n(You can make a copy of, or modify, this frame)"
        n73 = call <vilib>:"Add State(s) to Queue__jki_lib_state_machine.vi"("State(s) in (\"\")"=w194) -> ("States Out"=w193:string)  [unwired: 14 in]
      }
      frame #18 {
        # "Sets the list of states to execute on vi startup in the first string and  the list of states to execute on each loop\nin the second string"
        n74 = local write "Tab Control"(0) -> ()
        n75 = call <vilib>:"Add State(s) to Queue__jki_lib_state_machine.vi"("State(s) in Front (\"\")"="Main: Read Expt Configs\nMain: Get Expt name\nMain: Read Expt Config\nGet List of Axis Names\nGet Default Y Axis\nMain: Set Panel Postion\nMain: Get Device Configs\nPlot", "State(s) in (\"\")"=w200) -> ("States Out"=w199:string)  [unwired: 13 in]
      }
      frame #19 {
        # "Gets experimental configuration filenames. These files contain information specific to an experiment. Eg TREX expt\nfile would have all the devices that need to startup and their default variable values."
        n76 = call "preset SQL Queries.vi"("error in (no error)"=w202, "Preset Query"=Preset_Query_Enum."Get Expt names") -> ("error out"=w201:errorcluster, "1st column"=w203:string[])  [unwired: 7 in, 1 out]
        n77 = call "array to strings and values for ring.vi"("list of variables"=w203) -> ("Array"=w207:cluster{"String":string, i32}[])
        n78 = property on="Experiment" class="Ring (strict)"("StringsAndValues[]"=w207) -> ()  [unwired: 2 in, 2 out]
        n79 = Bundle By Name(cluster=w206, "Expt Config Files"=w203) -> (w205:T10)
        n80 = call <vilib>:"Add State(s) to Queue__jki_lib_state_machine.vi"("State(s) in (\"\")"=w209) -> ("States Out"=w208:string)  [unwired: 14 in]
      }
      frame #20 {
        # "Increments scan #, resets shot number and sends list of states to execute at the start of a scan. Only does this\nif variable for scan is numeric."
        n81 = Unbundle By Name(w215) -> ("Expt Config Files"=w213:string[])
        n82 = Index Array(array=w213, index="Experiment") -> (element=w211:string)
        n83 = Bundle By Name(cluster=w215, "Experiment name"=w211) -> (w214:T10)
        n84 = call <vilib>:"Add State(s) to Queue__jki_lib_state_machine.vi"("State(s) in (\"\")"=w217) -> ("States Out"=w216:string)  [unwired: 14 in]
      }
      frame #21 {
        # "todo. get rid of the copy of parameters"
        # "Reads the configuration for a particular experiment. eg TREX default would save spectrum mode image and\nget back centroid etc."
        n85 = Unbundle By Name(w231) -> ("Experiment name"=w222:string)
        n86 = call "preset SQL Queries.vi"("error in (no error)"=w221, "Device/Devicetype name"=w222, "Preset Query"=Preset_Query_Enum."Get expt devices with data to get") -> ("error out"=w229:errorcluster, "data"=w226:string[][])  [unwired: 6 in, 1 out]
        n87 = Delete From Array(array=w226, index (row)=0) -> (array with subset deleted=w228:string[][])  [unwired: 2 in, 1 out]
        n88 = Index Array(array=w228, index (col)=0 ("disabled index (col)")) -> (element=w219:string[])  [unwired: 1 in]
        "devices to get data from" <- w219
        n89 = call "preset SQL Queries.vi"("error in (no error)"=w229, "Device/Devicetype name"=w222, "Preset Query"=Preset_Query_Enum."Get expt devices and variables (with data to get)") -> ("error out"=w220:errorcluster, "data"=w218:string[][])  [unwired: 6 in, 1 out]
        "parameters to get" <- w218
        n90 = Bundle By Name(cluster=w231, "expt config file array"=w218, "ScanData to receive"=w218, "Device Names for scan data"=w219) -> (w230:T10)
        n91 = call <vilib>:"Add State(s) to Queue__jki_lib_state_machine.vi"("State(s) in (\"\")"=w233) -> ("States Out"=w232:string)  [unwired: 14 in]
      }
      frame #22 {
        # "Increments scan #, resets shot number and sends list of states to execute at the start of a scan. Only does this\nif variable for scan is numeric."
        n92 = Unbundle By Name(w235) -> ("ScanData to receive"=w241:string[][])
        n93 = Index Array(array=w241, index (col) #1=0 ("disabled index (col)"), index (col) #2=1 ("index (col)")) -> (element #1=w238:string[], element #2=w237:string[])  [unwired: 2 in]
        n94 = for {
          tunnel: w238 -> [w247] mode=indexing
          tunnel: w237 -> [w246] mode=indexing
          tunnel: [w245] -> w236 mode=indexing
          n95 = Concatenate Strings(w247, " " ("string"), w246) -> (w245:string)
        }
        "Axis Name List" <- w236
        n96 = Bundle By Name(cluster=w235, "Data titles from config array"=w236) -> (w234:T10)
        n97 = call <vilib>:"Add State(s) to Queue__jki_lib_state_machine.vi"("State(s) in (\"\")"=w244) -> ("States Out"=w243:string)  [unwired: 14 in]
      }
      frame #23 {
        # "todo. Fix above since changed to Database"
        # "TODO re-enable"
        # "Increments scan #, resets shot number and sends list of states to execute at the start of a scan. Only does this\nif variable for scan is numeric."
        n98 = Unbundle By Name(w255) -> ("expt config file array"=w257:string[][])
        n99 = String To IP() -> (0:w260:u32)  [unwired: 1 in]
        n100 = IP To String(1:TRUE ("dot notation? (F)"), 2:w260) -> (0:w259:string)
        "MY IP" <- w259
        n101 = Index Array(array=w257, index (col)=8 ("disabled index (col)")) -> (element=w262:string[])  [unwired: 1 in]
        n102 = call-poly <userlib>:"Search Array__ogtk.vi"("Array"=w262, "Element Data"=w259) -> ("Indices of Elements"=w258:i32[])  [unwired: 7 in]
        n103 = Index Array(array=w258) -> (element=w256:i32)  [unwired: 1 in]
        n104 = Index Array(array=w257, index (row)=w256) -> (element=w254:string[])  [unwired: 1 in]
        n105 = Index Array(array=w254) -> (element #1=w253:string, element #2=w251:string)  [unwired: 2 in]
        n106 = Concatenate Strings(w253, " " ("string"), w251) -> (w249:string)
        "Y Axis Default name" <- w249
        n107 = property on="Y Axis" class="Ring (strict)"() -> ("Strings []"=w250:string[])  [unwired: 2 in, 2 out]
        n108 = call <vilib>:"Add State(s) to Queue__jki_lib_state_machine.vi"("State(s) in (\"\")"=w266) -> ("States Out"=w265:string)  [unwired: 14 in]
        n109 = disable-structure shown="Disabled" {
          disable-tunnel: w250 -> [w269 _]
          disable-tunnel: w249 -> [w268 _]
          frame #0 {
            n110 = Search 1D Array(1D array=w269, element=w268) -> (index of element=w267:i32)  [unwired: 1 in]
            n111 = local write "Y Axis"(w267) -> ()
          }
          frame #1 {
          }
        }
      }
      frame #24 {
        # "Reads the configuration for a particular experiment. eg TREX default would save spectrum mode image and\nget back centroid etc."
        n112 = control-ref of="This VI"() -> (w286:refnum<vi>)
        n113 = property class="VI"(reference=w286) -> (reference out=w281:refnum<vi>, error out=w279:errorcluster, "Panel"=w288:refnum<vi>)  [unwired: 1 in]
        n114 = property on="Tab Control" class="TabCtl (strict)"() -> ("PaneWidth"=w275:u32, "PaneHeight"=w274:u32)  [unwired: 2 in, 2 out]
        n115 = Add(x=w274, y=u32 25) -> (x+y=w272:u32)
        n116 = Add(x=u32 2, y=w275) -> (x+y=w273:u32)
        n117 = property class="Pnl"(reference=w288, error in=w279) -> (reference out=w282:refnum<vi>, error out=w278:errorcluster, "Position"=→"Position":T2, "Panes[]"=w285:refnum<vi>[])
        n118 = Index Array(array=w285) -> (element=w284:refnum<vi>)  [unwired: 1 in]
        n119 = property class="Pane"(reference=w284, error in=w278) -> (error out=w277:errorcluster, "Origin"=w283:T11)  [unwired: 1 out]
        "Position 2" <- w283
        n120 = Add(x="Top", y=w272) -> (x+y=w293:u32)
        n121 = Add(x="Left", y=w273) -> (x+y=w290:u32)
        n122 = property class="Pnl"(reference=w282, error in=w277, "Position"=w283) -> (error out=w276:errorcluster)  [unwired: 1 out]
        n123 = Bundle By Name(cluster=T7 {"Left"=0, "Top"=0, "Right"=0, "Bottom"=0} ("Front Panel Window:Panel Bounds"), "Left"="Left", "Top"="Top", "Right"=w290, "Bottom"=w293) -> (w280:T7)
        n124 = property class="VI"(reference=w281, error in=w276, "Front Panel.PanelBounds"=w280) -> ()  [unwired: 2 out]
        n125 = call <vilib>:"Add State(s) to Queue__jki_lib_state_machine.vi"("State(s) in (\"\")"=w297) -> ("States Out"=w296:string)  [unwired: 14 in]
      }
      frame #25 {
        # "Reads the configuration for a particular experiment. eg TREX default would save spectrum mode image and\nget back centroid etc."
        n126 = call "preset SQL Queries.vi"("Preset Query"=Preset_Query_Enum."Get all devices basic properties") -> ("data"=w298:string[][])  [unwired: 8 in, 2 out]
        "All Devices Core Info" <- w298
        n127 = Bundle By Name(cluster=w300, "All Devices Core Info"=w298) -> (w301:T10)
        n128 = call <vilib>:"Add State(s) to Queue__jki_lib_state_machine.vi"("State(s) in (\"\")"=w304) -> ("States Out"=w303:string)  [unwired: 14 in]
      }
      frame #26 {
        # "Your code here.\n(You can make a copy of, or modify, this frame)"
        n129 = disable-structure shown="Enabled" {
          disable-tunnel: w305 -> [_ w318]
          frame #0 {
            n130 = TDMS Open(6:FALSE ("disable buffering (T)"), 7:enum16{"1.0", "2.0"}."1.0" ("file format version (2.0)"), 10:T8."open" ("operation")) -> ()  [unwired: 3 in, 2 out]
            n131 = TDMS Close() -> ()  [unwired: 2 in, 1 out]
          }
          frame #1 {
            n132 = Unbundle By Name(w318) -> ("TDMS file path"=w316:path)
            "TDMS file path" <- w316
            n133 = Select(t="file path", s="FilePath", f=w316) -> (s? t:f=w314:path)
            "Path used" <- w314
            n134 = call <vilib>:"Check if File or Folder Exists.vi"("path"=w314) -> ("file or folder exists?"=w313:bool, "dup path"=w312:path)  [unwired: 8 in, 1 out]
            n135 = case shown="True" w313 {
              tunnel: w312 -> [_ w319]
              frame #0 {
              }
              frame #1 {
                n136 = call "Read TDMS - LOASIS scan data.vi"("file path"=w319) -> ("device data Spreadsheet format"=w320:string[][])  [unwired: 10 in]
                "device data Spreadsheet format" <- w320
                n137 = stacked-sequence {
                  tunnel: w320 -> [w323 w331 _ _ _ _]
                  frame #0 {
                    n138 = Index Array(array=w323, index (row)=0) -> (element=w321:string[])  [unwired: 1 in]
                    n139 = property on="X Axis" class="Ring (strict)"("Strings []"=w321) -> ()  [unwired: 2 in, 2 out]
                    n140 = property on="Y Axis" class="Ring (strict)"("Strings []"=w321) -> ()  [unwired: 2 in, 2 out]
                  }
                  frame #1 {
                    n141 = control-ref of="XY Graph"() -> (w329:refnum<vi>)
                    n142 = control-ref of="Y Axis 2"() -> (w328:refnum<vi>)
                    n143 = control-ref of="Y Axis"() -> (w327:refnum<vi>)
                    n144 = control-ref of="X Axis"() -> (w326:refnum<vi>)
                    n145 = Bundle By Name(cluster=T9 {"Ring Refnum x"=refnum, "Ring Refnum y"=refnum, "Ring Refnum y 2"=refnum, "XY Graph Refnum"=refnum} ("Cluster"), "Ring Refnum x"=w326, "Ring Refnum y"=w327, "Ring Refnum y 2"=w328, "XY Graph Refnum"=w329) -> (w324:T9)
                    n146 = call "Select axes.vi"("Cluster"=w324, "output array"=w331) -> ("XY Graph"=→"xy graph":cluster{dbl[], dbl[]}[])  [unwired: 4 in, 2 out]
                  }
                  frame #2 {
                    # "TODO re-enable"
                    n147 = disable-structure shown="Disabled" {
                      frame #0 {
                        n148 = local read "x axis name"() -> (w333:string)
                        n149 = property on="X Axis" class="Ring (strict)"() -> ("Strings []"=w334:string[])  [unwired: 2 in, 2 out]
                        n150 = Search 1D Array(1D array=w334, element=w333) -> (index of element=w332:i32)  [unwired: 1 in]
                        n151 = local write "X Axis"(w332) -> ()
                      }
                      frame #1 {
                      }
                    }
                  }
                  frame #3 {
                    n152 = case shown="True" "Auto Interval" {
                      frame #0 {
                      }
                      frame #1 {
                        n153 = local read "xy graph"() -> (w338:cluster{dbl[], dbl[]}[])
                        n154 = Index Array(array=w338) -> (element=w336:cluster{dbl[], dbl[]})  [unwired: 1 in]
                        n155 = Unbundle(w336) -> (w337:dbl[])  [unwired: 1 out]
                        n156 = Array Max & Min(array=w337) -> (max value=w340:dbl, min value=w341:dbl)  [unwired: 2 out]
                        n157 = Subtract(x=w340, y=w341) -> (x-y=w342:dbl)
                        n158 = Divide(x=w342, y=10.0) -> (x/y=w339:dbl)
                        n159 = local write "Interval"(w339) -> ()
                      }
                    }
                  }
                  frame #4 {
                    n160 = property on="xy graph" class="XYGraph (strict)"() -> ("XScale.NameLbl.Text"=w345:string, "YScale.NameLbl.Text"=w344:string)  [unwired: 2 in, 2 out]
                    n161 = property on="xy graph" class="XYGraph (strict)"("XScale.NameLbl.Text"=w345, "YScale.NameLbl.Text"=w344) -> ()  [unwired: 2 in, 2 out]
                  }
                  frame #5 {
                    n162 = disable-structure shown="Enabled" {
                      frame #0 {
                        # "todo. use multiple bin"
                        n163 = local read "xy graph"() -> (w346:cluster{dbl[], dbl[]}[])
                        n164 = Index Array(array=w346) -> (element=w347:cluster{dbl[], dbl[]})  [unwired: 1 in]
                        n165 = Unbundle(w347) -> (w352:dbl[])  [unwired: 1 out]
                        n166 = Array Size(array=w352) -> (size(s)=w353:i32)
                        n167 = Not Equal To 0?(x=w353) -> (x != 0?=w350:bool)
                        n168 = Not Equal To 0?(x="Interval") -> (x != 0?=w349:bool)
                        n169 = And(x=w350, y=w349) -> (x .and. y?=w348:bool)
                        n170 = case shown="True" w348 {
                          tunnel: w346 -> [_ w358]
                          tunnel: "Interval" -> [_ w354]
                          frame #0 {
                          }
                          frame #1 {
                            n171 = call "bin multiple xy graphs-b.vi"("Error Bar Type"="Error Bar Type", "interval"=w354, "FIXED X INTERVAL?"="Fixed Interval", "parameter 2,3,4 vs 1"=w358) -> ("Array"=→"xy graph":cluster{"y vector":dbl[], "avg optspec":dbl[]}[])  [unwired: 1 out]
                          }
                        }
                      }
                      frame #1 {
                      }
                    }
                  }
                }
              }
            }
          }
        }
        n172 = call <vilib>:"Add State(s) to Queue__jki_lib_state_machine.vi"("State(s) in (\"\")"=w308) -> ("States Out"=w307:string)  [unwired: 14 in]
      }
      frame #27 {
        # "Your code here.\n(You can make a copy of, or modify, this frame)"
        n173 = call <vilib>:"Add State(s) to Queue__jki_lib_state_machine.vi"("State(s) in (\"\")"=w362) -> ("States Out"=w361:string)  [unwired: 14 in]
      }
    }
  }
  n174 = String To IP(1:"234.5.6.9" ("Multicast Address")) -> (0:w10:u32)
  n175 = call-poly <vilib>:"UDP Multicast Open.vi"("multicast addr"=w10, "port"=58432 ("Port")) -> ("error out"=w4:errorcluster, "connection ID"=w8:refnum<k16>)  [unwired: 7 in, 1 out]
  n176 = call "Plotter stop FGV.vi"("Function"=enum16{"Read", "Write", "Clear"}."Clear") -> ("error out"=w1:errorcluster)  [unwired: 9 in, 1 out]
  n177 = while {
    tunnel: w8 -> [w385]
    tunnel: [w383] -> w7
    tunnel: [w382] -> w6
    tunnel: w4 -> [w376]
    tunnel: w1 -> [w373]
    stop <- w375 stop-if-true
    n178 = call "Plotter stop FGV.vi"("error in"=w373, "Function"=enum16{"Read", "Write", "Clear"}."Read") -> ("Stop out"=w375:bool)  [unwired: 8 in, 1 out]
    n179 = UDP Read(connection ID=w385, timeout ms (25000)=100, 8:w376) -> (data out=w363:string, error out=w384:errorcluster, 3:w383:refnum<k16>)  [unwired: 3 out]
    "Mcast Data" <- w363
    n180 = call "no timeout error.vi"("error in (no error)"=w384) -> ("error out"=w382:errorcluster)
    n181 = String Subset(string=w363, length (rest)=4 ("length (rest)")) -> (substring=w370:string)  [unwired: 1 in]
    n182 = String Subset(string=w363, offset (0)=6) -> (substring=w368:string)  [unwired: 1 in]
    n183 = call "string to 1d array.vi"("delimiter (Tab)"=">>", "string"=w363) -> ("Array of Strings"=w380:string[])  [unwired: 9 in]
    n184 = Equal?(x="Path" ("y"), y=w370) -> (x = y?=w366:bool)
    n185 = Index Array(array=w380, index #1=0 ("index")) -> (element #1=w378:string, element #2=w364:string, element #3=w365:string)  [unwired: 2 in]
    n186 = Equal?(x="ScanStart", y=w378) -> (x = y?=w367:bool)
    n187 = case shown="True" w366 {
      tunnel: w368 -> [_ w387]
      frame #0 {
      }
      frame #1 {
        n188 = property on="Mcast Path Data" class="Str"("Val(Sgnl)"=w387) -> ()  [unwired: 2 in, 2 out]
        "Mcast Path Data" <- w387
      }
    }
    n189 = case shown="True" w367 {
      tunnel: w365 -> [_ w389]
      tunnel: w364 -> [_ w388]
      frame #0 {
      }
      frame #1 {
        n190 = property on="ScanStart ExptName" class="Str"("Val(Sgnl)"=w388) -> ()  [unwired: 2 in, 2 out]
        "x axis name" <- w389
        "ScanStart ExptName" <- w388
      }
    }
  }
  n191 = UDP Close(connection ID=w7, 8:w6) -> (error out=→"UDP Mcast Error":errorcluster)  [unwired: 1 out]
